vi "srednia_rekurencyjnie_(SubVI).vi"(9 "N":i32, 10 "œr N-1":dbl, 11 "Gaussian white noise":dbl) -> (3 "œrednia":dbl)   [LabVIEW 2025]
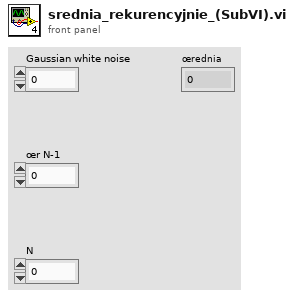
[diagram p1: front panel]
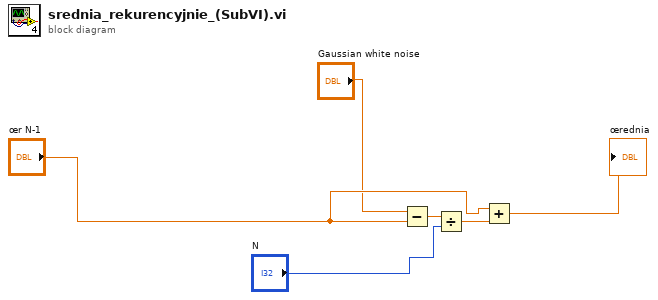
[diagram p0: block diagram]
diagram:
  n1 = Subtract(x="Gaussian white noise", y="œr N-1") -> (x-y=w2:dbl)
  n2 = Divide(x=w2, y="N") -> (x/y=w4:dbl)
  n3 = Add(x="œr N-1", y=w4) -> (x+y=→"œrednia":dbl)
